vi "waveformpreparearp.vi"(9 "1762 Sweep length (units of .1 us)":i32) -> (3 "digital waveform out 2":digitalwaveform(waveform)={"t0"=timestamp(0 s since 1904-01-01), "dt"=1e-06, "Y"={"transitions"=[0, 10001], "data"=[[1, 1, 0, 0], [0, 0, 0, 0]]}, "error"={"status"=FALSE, "code"=37421928, "source"=""}})   [LabVIEW 2012]
uses:
  <vilib>/Waveform/DWDTOps.llb/Digital Pattern Generator (Single Value).vi
  <vilib>/Waveform/DWDTOps.llb/DWDT Append Digital Samples.vi
panel:
  out "out":digitalwaveform(waveform)={"t0"=timestamp(0 s since 1904-01-01), "dt"=0.0, "Y"={"transitions"=[], "data"=[]}, "error"={"status"=FALSE, "code"=37421928, "source"=""}}
  out "Mixed Signal Graph":digitalwaveform(graph)
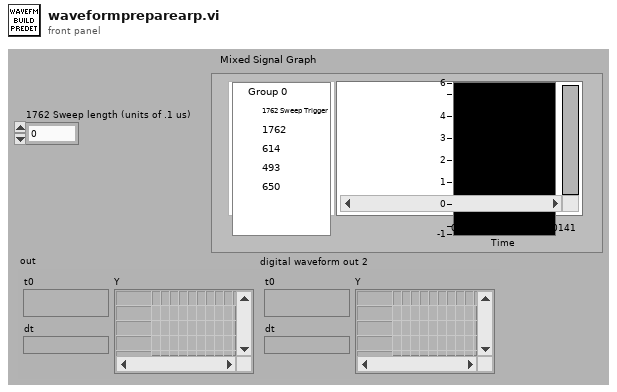
[diagram p1: front panel]
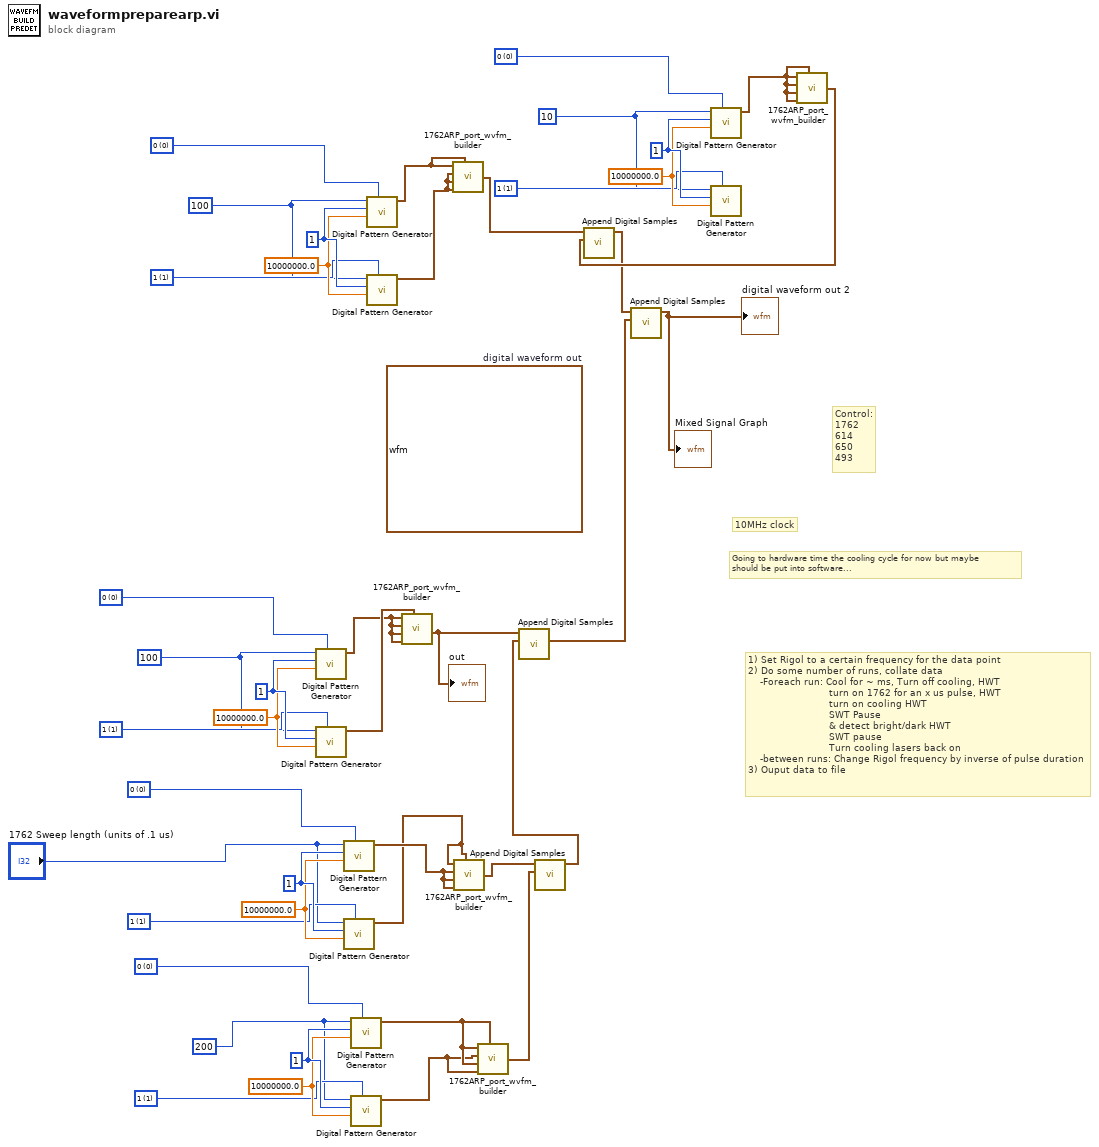
[diagram p0: block diagram]
diagram:
  w7 = u32 10 ("number of samples")
  w11 = u8 0 items=["0", "1", "Z", "L", "H", "X", "T", "V"] ("value")
  w10 = u32 1 ("number of signals")
  w8 = u8 1 items=["0", "1", "Z", "L", "H", "X", "T", "V"] ("value")
  w9 = 10000000.0 ("rate")
  w12 = u32 100 ("number of samples")
  w16 = u8 0 items=["0", "1", "Z", "L", "H", "X", "T", "V"] ("value")
  w15 = u32 1 ("number of signals")
  w13 = u8 1 items=["0", "1", "Z", "L", "H", "X", "T", "V"] ("value")
  w14 = 10000000.0 ("rate")
  w24 = u32 100 ("number of samples")
  w29 = u32 200 ("number of samples")
  w33 = u8 0 items=["0", "1", "Z", "L", "H", "X", "T", "V"] ("value")
  w32 = u32 1 ("number of signals")
  w30 = u8 1 items=["0", "1", "Z", "L", "H", "X", "T", "V"] ("value")
  w31 = 10000000.0 ("rate")
  w38 = u8 0 items=["0", "1", "Z", "L", "H", "X", "T", "V"] ("value")
  w37 = u32 1 ("number of signals")
  w35 = u8 1 items=["0", "1", "Z", "L", "H", "X", "T", "V"] ("value")
  w36 = 10000000.0 ("rate")
  w43 = u8 0 items=["0", "1", "Z", "L", "H", "X", "T", "V"] ("value")
  w42 = u32 1 ("number of signals")
  w40 = u8 1 items=["0", "1", "Z", "L", "H", "X", "T", "V"] ("value")
  w41 = 10000000.0 ("rate")
  (unwired) digitalwaveform {"t0"=timestamp(0 s since 1904-01-01), "dt"=1e-07, "Y"={"transitions"=[0, 200, 210], "data"=[[1, 1, 1, 0, 0], [0, 0, 0, 0, 0], [0, 0, 0, 0, 0]]}, "error"={"status"=FALSE, "code"=37421928, "source"=""}}  # digital waveform out
  # "Going to hardware time the cooling cycle for now but maybe\nshould be put into software..."
  # "10MHz clock"
  # "Control:\n1762\n614\n650\n493"
  # "1) Set Rigol to a certain frequency for the data point\n2) Do some number of runs, collate data\n    -Foreach run: Cool for ~ ms, Turn off cooling, HWT\n                           turn on 1762 for an x us pulse, HWT\n                           turn on cooling HWT\n                           SWT Pause\n                           & detect bright/dark HWT\n                           SWT pause\n                           Turn cooling lasers back on \n    -between runs: Change Rigol frequency by inverse of pulse duration\n3) Ouput data to file"
  n1 = call-poly <vilib>:"Digital Pattern Generator.vi"("value"=w43, "sample rate"=w41, "number of signals"=w42, "number of samples"=w24) -> ("digital waveform"=w25:digitalwaveform)  [unwired: 6 in, 1 out]
  n2 = call-poly <vilib>:"Digital Pattern Generator.vi"("value"=w40, "sample rate"=w41, "number of signals"=w42, "number of samples"=w24) -> ("digital waveform"=w26:digitalwaveform)  [unwired: 6 in, 1 out]
  n3 = call-poly <vilib>:"Digital Pattern Generator.vi"("value"=w38, "sample rate"=w36, "number of signals"=w37, "number of samples"="1762 Sweep length (units of .1 us)") -> ("digital waveform"=w23:digitalwaveform)  [unwired: 6 in, 1 out]
  n4 = call-poly <vilib>:"Digital Pattern Generator.vi"("value"=w35, "sample rate"=w36, "number of signals"=w37, "number of samples"="1762 Sweep length (units of .1 us)") -> ("digital waveform"=w22:digitalwaveform)  [unwired: 6 in, 1 out]
  n5 = call-poly <vilib>:"Digital Pattern Generator.vi"("value"=w33, "sample rate"=w31, "number of signals"=w32, "number of samples"=w29) -> ("digital waveform"=w18:digitalwaveform)  [unwired: 6 in, 1 out]
  n6 = call-poly <vilib>:"Digital Pattern Generator.vi"("value"=w30, "sample rate"=w31, "number of signals"=w32, "number of samples"=w29) -> ("digital waveform"=w17:digitalwaveform)  [unwired: 6 in, 1 out]
  n7 = call-poly <vilib>:"Digital Pattern Generator.vi"("value"=w16, "sample rate"=w14, "number of signals"=w15, "number of samples"=w12) -> ("digital waveform"=w5:digitalwaveform)  [unwired: 6 in, 1 out]
  n8 = call-poly <vilib>:"Digital Pattern Generator.vi"("value"=w13, "sample rate"=w14, "number of signals"=w15, "number of samples"=w12) -> ("digital waveform"=w6:digitalwaveform)  [unwired: 6 in, 1 out]
  n9 = call "1762ARP_port_wvfm_builder.vi"("1762 Sweep Trig"=w25, "493"=w25, "614"=w25, "650"=w25, "1762"=w26) -> ("out"=w27:digitalwaveform)
  "out" <- w27
  n10 = call "1762ARP_port_wvfm_builder.vi"("1762 Sweep Trig"=w5, "493"=w6, "614"=w6, "650"=w6, "1762"=w5) -> ("out"=w3:digitalwaveform)
  n11 = call "1762ARP_port_wvfm_builder.vi"("1762 Sweep Trig"=w22, "493"=w23, "614"=w23, "650"=w23, "1762"=w22) -> ("out"=w21:digitalwaveform)
  n12 = call "1762ARP_port_wvfm_builder.vi"("1762 Sweep Trig"=w18, "493"=w17, "614"=w18, "650"=w17, "1762"=w18) -> ("out"=w20:digitalwaveform)
  n13 = call-poly <vilib>:"Append Digital Samples.vi"("digital waveform B"=w20, "digital waveform A"=w21) -> ("digital waveform out"=w28:digitalwaveform)  [unwired: 8 in, 1 out]
  n14 = call-poly <vilib>:"Append Digital Samples.vi"("digital waveform B"=w28, "digital waveform A"=w27) -> ("digital waveform out"=w34:digitalwaveform)  [unwired: 8 in, 1 out]
  n15 = call-poly <vilib>:"Digital Pattern Generator.vi"("value"=w11, "sample rate"=w9, "number of signals"=w10, "number of samples"=w7) -> ("digital waveform"=w4:digitalwaveform)  [unwired: 6 in, 1 out]
  n16 = call-poly <vilib>:"Digital Pattern Generator.vi"("value"=w8, "sample rate"=w9, "number of signals"=w10, "number of samples"=w7) -> ()  [unwired: 6 in, 2 out]
  n17 = call "1762ARP_port_wvfm_builder.vi"("1762 Sweep Trig"=w4, "493"=w4, "614"=w4, "650"=w4, "1762"=w4) -> ("out"=w2:digitalwaveform)
  n18 = call-poly <vilib>:"Append Digital Samples.vi"("digital waveform B"=w2, "digital waveform A"=w3) -> ("digital waveform out"=w1:digitalwaveform)  [unwired: 8 in, 1 out]
  n19 = call-poly <vilib>:"Append Digital Samples.vi"("digital waveform B"=w34, "digital waveform A"=w1) -> ("digital waveform out"=→"Mixed Signal Graph" →"digital waveform out 2":digitalwaveform)  [unwired: 8 in, 1 out]
